vi "Linker.Find Tests and Suites.vi"(11 "Linker:Read Info From File":T2(array[cluster])) -> (1 "All VIs defining a Test Runner":path[](array[path]), 2 "All VIs defining a suite":path[](array[path]), 3 "All VIs defining a test (excluding those defining a suite)":path[](array[path]))   [LabVIEW 2020, in "Caraya.lvlib" / "Test Runner.lvclass"]
uses:
  <vilib>/addons/_JKI Toolkits/Caraya/classes/Test Runner/Test Runner.lvclass
  <vilib>/Utility/lvfile.llb/LVFileType.ctl
  <vilib>/Utility/lvfile.llb/NI_FileType.lvlib
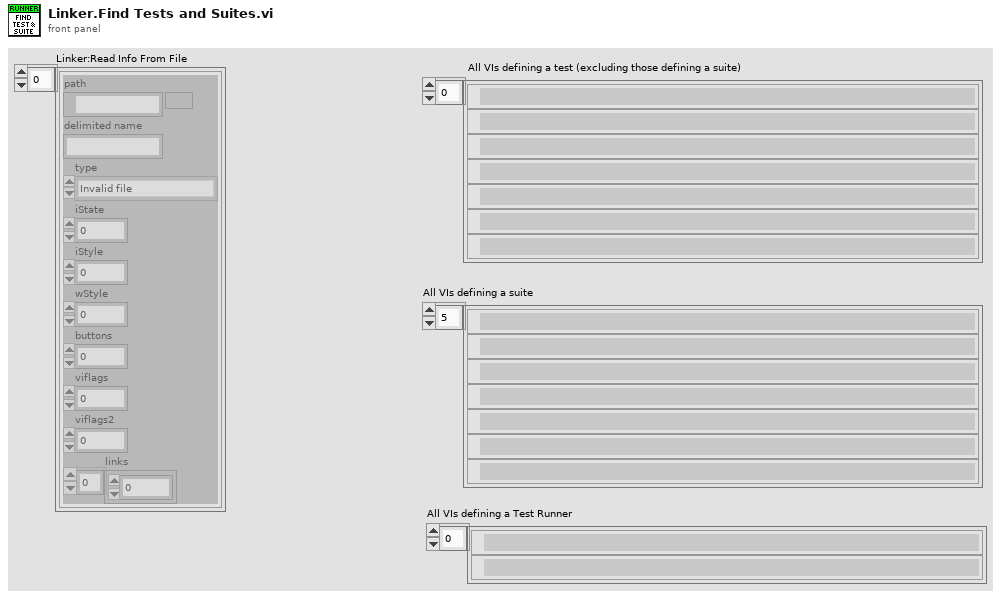
[diagram p1: front panel]
types:
  T1 = typedef "NI_FileType.lvlib/LVFileType.ctl" = enum32{"Invalid file", "Unknown type", "Instrument", "Control", "Polymorphic VI", "Project", "Library", "LVClass", "XControl", "XNode", "Shared library", ".NET assembly", "ActiveX interface", "CIN", "Run-time menu", "Palette menu", "Help file", "LLB", "XNode Edit Dependency", "Class Private Data Control", "Statechart", "MathScript .m file", "Ladder Diagram", "LVLibp", "XNode Build Dependency"}
  T2 = cluster{"path":path, "delimited name":string, "type":T1, "iState":u32, "iStyle":u16, "wStyle":u16, "buttons":u16, "viflags":u32, "viflags2":u32, "links":u32[]}[]
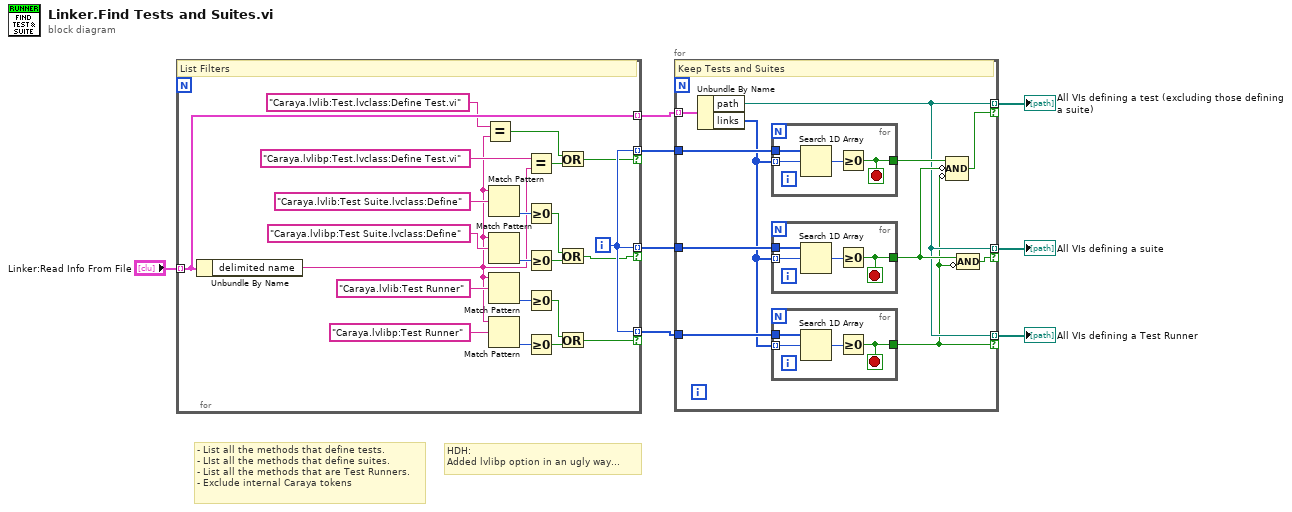
[diagram p0: block diagram]
diagram:
  # "HDH:\nAdded lvlibp option in an ugly way..."
  # "- List all the methods that define tests.\n- LIst all the methods that define suites.\n- List all the methods that are Test Runners.\n- Exclude internal Caraya tokens"
  n1 = for {
    tunnel: "Linker:Read Info From File" -> [w27] mode=indexing
    tunnel: [w22] -> w8 mode=indexing if=w11
    tunnel: [w22] -> w7 mode=indexing if=w10
    tunnel: [w27] -> w6 mode=indexing
    tunnel: [w22] -> w2 mode=indexing if=w9
    i -> [w22]
    # "List Filters"
    n2 = Unbundle By Name(w27) -> ("delimited name"=w13:string)
    n3 = Equal?(x="Caraya.lvlib:Test.lvclass:Define Test.vi" ("pattern"), y=w13) -> (x = y?=w29:bool)
    n4 = Match Pattern(string=w13, regular expression="Caraya.lvlib:Test Suite.lvclass:Define" ("pattern")) -> (offset past match=w30:i32)  [unwired: 1 in, 3 out]
    n5 = Match Pattern(string=w13, regular expression="Caraya.lvlibp:Test Suite.lvclass:Define" ("pattern")) -> (offset past match=w17:i32)  [unwired: 1 in, 3 out]
    n6 = Match Pattern(string=w13, regular expression="Caraya.lvlib:Test Runner" ("pattern")) -> (offset past match=w23:i32)  [unwired: 1 in, 3 out]
    n7 = Match Pattern(string=w13, regular expression="Caraya.lvlibp:Test Runner" ("pattern")) -> (offset past match=w15:i32)  [unwired: 1 in, 3 out]
    n8 = Equal?(x="Caraya.lvlibp:Test.lvclass:Define Test.vi" ("pattern"), y=w13) -> (x = y?=w19:bool)
    n9 = Greater Or Equal To 0?(x=w30) -> (x >= 0?=w28:bool)
    n10 = Greater Or Equal To 0?(x=w17) -> (x >= 0?=w16:bool)
    n11 = Greater Or Equal To 0?(x=w23) -> (x >= 0?=w21:bool)
    n12 = Greater Or Equal To 0?(x=w15) -> (x >= 0?=w12:bool)
    n13 = Or(x=w29, y=w19) -> (x .or. y?=w11:bool)
    n14 = Or(x=w28, y=w16) -> (x .or. y?=w10:bool)
    n15 = Or(x=w21, y=w12) -> (x .or. y?=w9:bool)
  }
  n16 = for {
    tunnel: w6 -> [w37] mode=indexing
    tunnel: w8 -> [w41]
    tunnel: [w32] -> w4 mode=indexing if=w38
    tunnel: w7 -> [w40]
    tunnel: [w32] -> w3 mode=indexing if=w34
    tunnel: w2 -> [w36]
    tunnel: [w32] -> w1 mode=indexing if=w31
    # "Keep Tests and Suites"
    n17 = Unbundle By Name(w37) -> ("path"=w32:path, "links"=w35:u32[])
    n18 = for {
      tunnel: w41 -> [w53]
      tunnel: w35 -> [w52] mode=indexing
      tunnel: [w50] -> w39
      stop <- w50 stop-if-true
      n19 = Search 1D Array(1D array=w53, element=w52) -> (index of element=w51:i32)  [unwired: 1 in]
      n20 = Greater Or Equal To 0?(x=w51) -> (x >= 0?=w50:bool)
    }
    n21 = for {
      tunnel: w40 -> [w49]
      tunnel: w35 -> [w48] mode=indexing
      tunnel: [w46] -> w33
      stop <- w46 stop-if-true
      n22 = Search 1D Array(1D array=w49, element=w48) -> (index of element=w47:i32)  [unwired: 1 in]
      n23 = Greater Or Equal To 0?(x=w47) -> (x >= 0?=w46:bool)
    }
    n24 = for {
      tunnel: w36 -> [w45]
      tunnel: w35 -> [w44] mode=indexing
      tunnel: [w42] -> w31
      stop <- w42 stop-if-true
      n25 = Search 1D Array(1D array=w45, element=w44) -> (index of element=w43:i32)  [unwired: 1 in]
      n26 = Greater Or Equal To 0?(x=w43) -> (x >= 0?=w42:bool)
    }
    n27 = Compound Arithmetic op=AND(w39, invert w33, invert w31) -> (w38:bool)
    n28 = Compound Arithmetic op=AND(w33, invert w31) -> (w34:bool)
  }
  "All VIs defining a test (excluding those defining a suite)" <- w4
  "All VIs defining a suite" <- w3
  "All VIs defining a Test Runner" <- w1
